vi "FPGA with torque filterMain.vi"() -> ()   [LabVIEW 2018]
doc: "This VI reads all analogue data channels available at the fastest rate supported by the respective hardware and updates a memory address for when each measurement is available.\n\nAt a rate defined by the fastest module (NI 9237 - default of 12.5kHz) this memory is read, combined with the measurements from the 9237 module and written to the FIFO for communication to the RT machine.\n\nThe NI 9237 modeul therefore defines the nominal sampling rate of the system (with slower channels over-sampled).\n\nA time channel (in uSec) is provided with 0 referenced from the first acquisition of the NI 9237 module"
uses:
  <vilib>/LabVIEW Targets/FPGA/cRIO/shared/nicrio_ModuleControls/nicrio_cRIO-9237_DataRatesRing.ctl
  <vilib>/Platform/TimedLoop/XDataNode/timing_clust.ctl
  <vilib>/Platform/TimedLoop/XDataNode/nitl_modes.ctl
  <vilib>/Platform/TimedLoop/XDataNode/wakeup.ctl
  <vilib>/rvi/Emulation/niFpgaGetClockAttributes.vi
  <vilib>/rvi/Emulation/niFpgaSctlEmulationGetInTimedLoop.vi
  <vilib>/rvi/Emulation/niFpgaEmulationReportErrorSimple.vi
  <vilib>/rvi/Emulation/niFpgaProcessEmulError.vi
  <vilib>/rvi/eio/common/nirviEmuTemplatePropertySet_noerrors.vi
  <vilib>/rvi/eio/common/nirviEmuTemplateMethod_errors.vi
  <vilib>/rvi/interface/RandomDataEmulation/niFpgaRandomDataHandleErrors.vi
  <vilib>/rvi/Memory/Memory_Emulation/nirvimemoryFastEmulation.vi
  <vilib>/rvi/Memory/Memory_Emulation/nirvimemoryEmulation.vi
  <vilib>/rvi/Emulation/niFpgaEmulationIsFPGAContextNoSignature.vi
  <vilib>/rvi/DataTransferAndStorage/Container/Common/niFpgaContainerGetUniqueNameForEmu.vi
  <vilib>/rvi/errors/nirviReportUnexpectedCaseInternalError (U32).vi
  <vilib>/rvi/Emulation/niFpgaCriticalErrorInLSC.vi
  <vilib>/eio/EIOPropertyNode/EIOPropertyNode.xnode
  <vilib>/eio/EIONode/EIONode.xnode
  <vilib>/rvi/DataTransferAndStorage/Container/XNode/niFpgaContainer.xnode
  <vilib>/rvi/interface/RandomDataEmulation/nirviRandomDataFpgaReadWriteTemplate.vi
  <vilib>/platform/TimedLoop/XDataNode/XDataNode.xnode
  <vilib>/eio/EIOMethodNode/EIOMethodNode.xnode
  <vilib>/Platform/TimedLoop/XDataNode/XDNodeRunTimeDep.lvlib
  <vilib>/rvi/eio/common/nirviEmuTemplatePropertyGet_errors.vi
  <vilib>/rvi/eio/common/nirviEmuTemplatePropertyGet_noerrors.vi
  <vilib>/rvi/eio/common/nirviEmuTemplatePropertySet_errors.vi
panel:
  in  "Data Rate":T1=1 items=["50.000 kS/s (NI 9237)"=1, "25.000 kS/s (NI 9237)"=2, "16.667 kS/s (NI 9237)"=3, "12.500 kS/s (NI 9237)"=4, "10.000 kS/s (NI 9237)"=5, "8.333 kS/s (NI 9237)"=6, "7.143 kS/s (NI 9237)"=7, "6.250 kS/s (NI 9237)"=8, "5.556 kS/s (NI 9237)"=9, "5.000 kS/s (NI 9237)"=10, "4.545 kS/s (NI 9237)"=11, "4.167 kS/s (NI 9237)"=12, "3.846 kS/s (NI 9237)"=13, "3.571 kS/s (NI 9237)"=14, "3.333 kS/s (NI 9237)"=15, "3.125 kS/s (NI 9237)"=16, "2.941 kS/s (NI 9237)"=17, "2.778 kS/s (NI 9237)"=18, "2.632 kS/s (NI 9237)"=19, "2.500 kS/s (NI 9237)"=20, "2.381 kS/s (NI 9237)"=21, "2.273 kS/s (NI 9237)"=22, "2.174 kS/s (NI 9237)"=23, "2.083 kS/s (NI 9237)"=24, "2.000 kS/s (NI 9237)"=25, "1.923 kS/s (NI 9237)"=26, "1.852 kS/s (NI 9237)"=27, "1.786 kS/s (NI 9237)"=28, "1.724 kS/s (NI 9237)"=29, "1.667 kS/s (NI 9237)"=30, "1.613 kS/s (NI 9237)"=31]
  in  "torque filter":i16=-2
  in  "encoders offset":u32 caption="encoder offset @ 1Hz (ticks)"
  out "Total channel count":u32=61
  out "timestamp":u32
  out "FIFO full counter":i32
  in  "Safe Voltage":fxp<+/-,20,5>[](array[numeric])=[0.0, 0.0, 0.0, 0.0]
  in  "Safe Digital":bool[](array[boolean])=[FALSE, FALSE, FALSE, FALSE, FALSE, FALSE, FALSE, FALSE]
  in  "Voltage Out":fxp<+/-,20,5>[](array[numeric])=[0.0, 0.0, 0.0, 0.0]
  in  "Update Outputs":bool
  in  "Mod 8":bool[](array[boolean])=[FALSE, FALSE, FALSE, FALSE, FALSE, FALSE, FALSE, FALSE]
  out "E Stop":bool
  in  "Stop acquire":bool
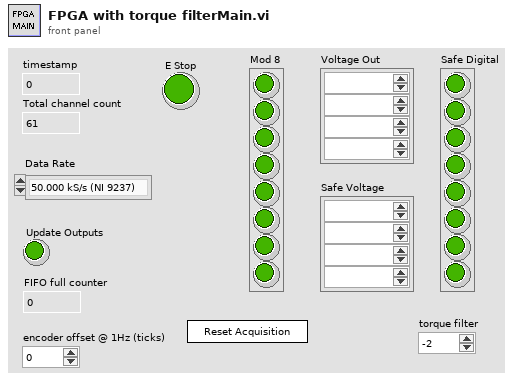
[diagram p1: front panel]
types:
  T1 = typedef "nicrio_cRIO-9237_DataRatesRing.ctl" = u8
  T2 = typedef "XDNodeRunTimeDep.lvlib/timing_clust.ctl" = cluster{"Expected End [f-1]":u64, "Actual End [f-1]":u64, "Finished Late? [f-1]":bool, "Expected End [i-1]":u64, "Actual End [i-1]":u64, "Finished Late? [i-1]":bool, "Expected Start [i]":u64, "Actual Start [i]":u64, "Expected Start [f]":u64, "Actual Start [f]":u64, "Source Name":string, "Structure Name":string, "Period":i64, "Deadline":i64, "Offset":i64, "Start":i64, "Priority":i32, "Timeout":i32, "Mode":T3, "Wakeup Reason":T4, "Error":errorcluster, "Source Type":string, "Secondary Source Type":string, "Global End Time":u64, "Global Start Time":u64, "Frame Duration":u64, "Iteration Duration":u64, "Assigned CPU":i32, "I/O Scan Engine Mode":u32}
  T3 = typedef "XDNodeRunTimeDep.lvlib/nitl_modes.ctl" = enum32{"No Change", "Process missed periods, maintain original phase", "Discard missed periods, maintain original phase", "Process missed periods, ignore original phase", "Discard missed periods, ignore original phase"}
  T4 = typedef "XDNodeRunTimeDep.lvlib/wakeup.ctl" = enum32{"Normal", "Aborted", "Asynchronous wakeup", "Timing source error", "Timed loop error", "Timeout"}
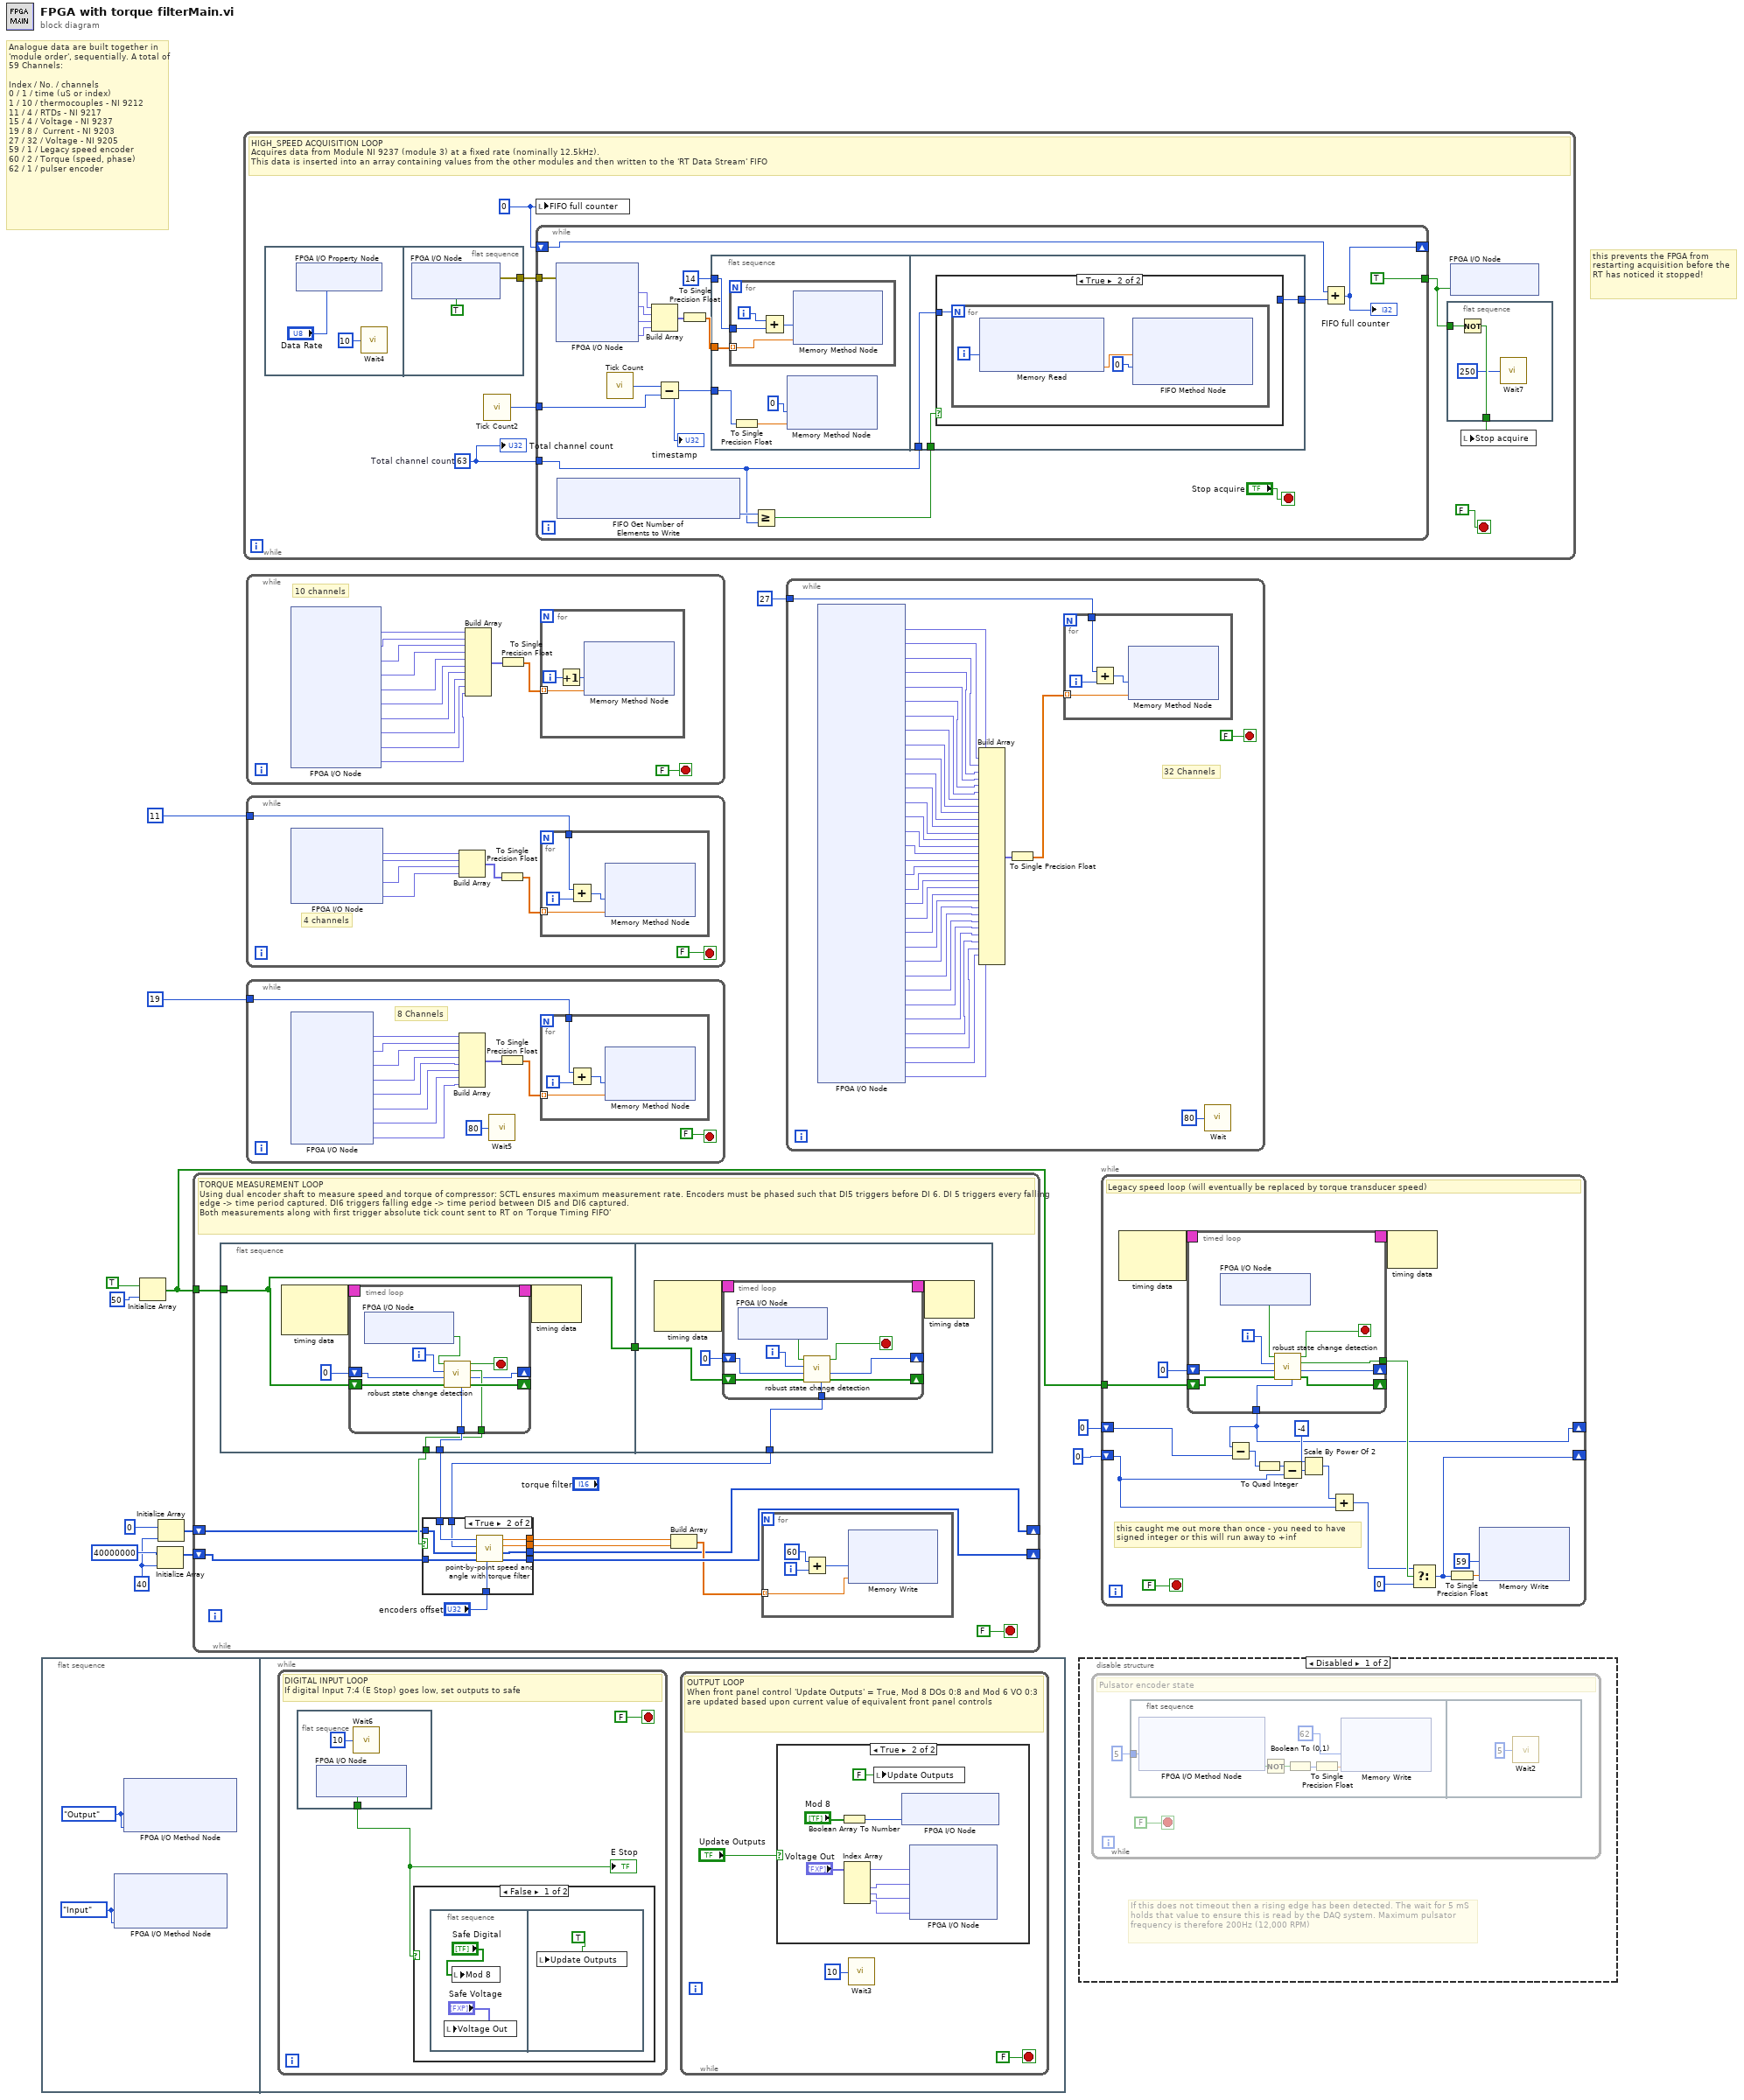
[diagram p0: block diagram]
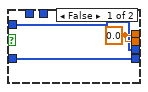
[diagram p5: hidden frame]
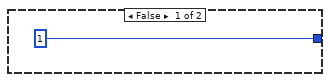
[diagram p6: hidden frame]
diagram:
  w3 = 40 ("dimension size")
  # "this prevents the FPGA from restarting acquisition before the RT has noticed it stopped!"
  # "Analogue data are built together in 'module order', sequentially. A total of 59 Channels:\n\nIndex / No. / channels\n0 / 1 / time (uS or index)\n1 / 10 / thermocouples - NI 9212\n11 / 4 / RTDs - NI 9217\n15 / 4 / Voltage - NI 9237\n19 / 8 /  Current - NI 9203\n27 / 32 / Voltage - NI 9205\n59 / 1 / Legacy speed encoder\n60 / 2 / Torque (speed, phase)\n62 / 1 / pulser encoder"
  n1 = flat-sequence {
    frame #0 {
      w14 = enum8{"No Change", "Input", "Output"}."Output" ("DIO 7:4")
      w15 = enum8{"No Change", "Input", "Output"}."Input" ("DIO 7:4")
      n2 = xnode "FPGA I/O Method Node"("DIO 7:4"=w15, "DIO 3:0"=w15) -> ()  [unwired: 1 in, 1 out]
      n3 = xnode "FPGA I/O Method Node"("DIO 7:4"=w14, "DIO 3:0"=w14) -> ()  [unwired: 1 in, 1 out]
    }
    frame #1 {
      n4 = while {
        stop <- FALSE stop-if-true
        # "DIGITAL INPUT LOOP\nIf digital Input 7:4 (E Stop) goes low, set outputs to safe"
        n5 = flat-sequence {
          tunnel: [w30] -> w27
          frame #0 {
            n6 = xnode "FPGA I/O Node"() -> ("Mod7/DIO4"=w30:bool)  [unwired: 1 in, 1 out]
            n7 = call "Wait6"("Count(uSec)"=u8 10) -> ()  [unwired: 1 out]
          }
        }
        n8 = case shown="False" w27 {
          frame False {
            n9 = flat-sequence {
              frame #0 {
                n10 = local write "Voltage Out"("Safe Voltage") -> ()
                n11 = local write "Mod 8"("Safe Digital") -> ()
              }
              frame #1 {
                n12 = local write "Update Outputs"(TRUE ("Update Outputs")) -> ()
              }
            }
          }
          frame True {
          }
        }
        "E Stop" <- w27
      }
      n13 = while {
        stop <- FALSE stop-if-true
        # "OUTPUT LOOP\nWhen front panel control 'Update Outputs' = True, Mod 8 DOs 0:8 and Mod 6 VO 0:3 are updated based upon current value of equivalent front panel controls"
        n14 = case shown="True" "Update Outputs" {
          frame False {
          }
          frame True {
            n15 = Boolean Array To Number(Boolean array="Mod 8") -> (number=w25:u8)
            n16 = Index Array(array="Voltage Out") -> (element #1=w23:fxp<+/-,20,5>, element #2=w22:fxp<+/-,20,5>, element #3=w21:fxp<+/-,20,5>, element #4=w20:fxp<+/-,20,5>)  [unwired: 4 in]
            n17 = local write "Update Outputs"(FALSE ("Update Outputs")) -> ()
            n18 = xnode "FPGA I/O Node"("Mod8/DIO7:0"=w25) -> ()  [unwired: 1 in, 1 out]
            n19 = xnode "FPGA I/O Node"("Mod6/AO0"=w23, "Mod6/AO1"=w22, "Mod6/AO2"=w21, "Mod6/AO3"=w20) -> ()  [unwired: 4 in, 4 out]
          }
        }
        n20 = call "Wait3"("Count(uSec)"=u16 10 ("Count(Ticks)")) -> ()  [unwired: 1 out]
      }
    }
  }
  n21 = Initialize Array(TRUE, 50 ("edge buffer size")) -> (w5:bool[])
  n22 = Initialize Array(u32 40000000 ("64bit integer"), w3) -> (w8:u32[])
  n23 = Initialize Array(0 ("64bit integer"), w3) -> (w1:i32[])
  n24 = while {
    shift-right: [w43] -> _
    shift-left: w8 -> [w44]
    tunnel: w5 -> [w38]
    shift-right: [w35] -> _
    shift-left: w1 -> [w36]
    stop <- FALSE stop-if-true
    # "TORQUE MEASUREMENT LOOP\nUsing dual encoder shaft to measure speed and torque of compressor: SCTL ensures maximum measurement rate. Encoders must be phased such that DI5 triggers before DI 6. DI 5 triggers every falling edge -> time period captured. DI6 triggers falling edge -> time period between DI5 and DI6 captured.\nBoth measurements along with first trigger absolute tick count sent to RT on 'Torque Timing FIFO'"
    n25 = flat-sequence {
      tunnel: [w67] -> w46
      tunnel: [w66] -> w39
      tunnel: w38 -> [w64]
      tunnel: [w64] -> w37
      tunnel: [w87] -> w45
      tunnel: w37 -> [w86]
      frame #0 {
        n26 = node-c288() -> (w69:T2)  [unwired: 2 in]
        n27 = timed-loop {
          timing: w69 -> [_]
          timing-out: [_] -> w68
          tunnel: [w73] -> w67
          tunnel: [w72] -> w66
          shift-right: [w76] -> _
          shift-left: w64 -> [w77]
          shift-right: [w70] -> _
          shift-left: i16 0 ("step") -> [w74]
          i -> [w75]
          stop <- w71 stop-if-true
          n28 = xnode "FPGA I/O Node"() -> ("Mod7/DIO0"=w78:bool)  [unwired: 1 in, 1 out]
          n29 = call "robust state change detection.vi"("history"=w77, "step"=w74, "tick"=w75, "New state"=w78) -> ("history out"=w76:bool[], "step out"=w70:i16, "edge detected"=w72:bool, "Stop?"=w71:bool, "tick"=w73:u32)  [unwired: 3 in]
        }
        n30 = node-c288(w68) -> ()  [unwired: 1 out]
      }
      frame #1 {
        n31 = node-c288() -> (w85:T2)  [unwired: 2 in]
        n32 = timed-loop {
          timing: w85 -> [_]
          timing-out: [_] -> w84
          shift-right: [w93] -> _
          shift-left: w86 -> [w94]
          tunnel: [w91] -> w87
          shift-right: [w88] -> _
          shift-left: i16 0 ("step") -> [w89]
          i -> [w90]
          stop <- w92 stop-if-true
          n33 = xnode "FPGA I/O Node"() -> ("Mod7/DIO1"=w95:bool)  [unwired: 1 in, 1 out]
          n34 = call "robust state change detection.vi"("history"=w94, "step"=w89, "tick"=w90, "New state"=w95) -> ("history out"=w93:bool[], "step out"=w88:i16, "Stop?"=w92:bool, "tick"=w91:u32)  [unwired: 3 in, 1 out]
        }
        n35 = node-c288(w84) -> ()  [unwired: 1 out]
      }
    }
    n36 = case shown="True" w39 {
      tunnel: w46 -> [_ w59]
      tunnel: w45 -> [_ w58]
      tunnel: w44 -> [w50 w57]
      tunnel: [w50 w56] -> w43
      tunnel: "encoders offset" -> [_ w55]
      tunnel: [w49 w54] -> w41
      tunnel: [w49 w53] -> w34
      tunnel: w36 -> [w48 w52]
      tunnel: [w48 w51] -> w35
      frame False {
        w49 = sgl 0.0 ("calculated speed (Hz)")
      }
      frame True {
        n37 = call "point-by-point speed and angle with torque filter.vi"("encoders offset"=w55, "speed history in"=w57, "torque history"=w52, "angle pulse"=w58, "speed pulse"=w59) -> ("speed history out"=w56:u32[], "torque history out"=w51:i32[], "calculated angle (degrees)"=w53:sgl, "calculated speed (Hz)"=w54:sgl)  [unwired: 2 in, 1 out]
      }
    }
    n38 = Build Array(w41, w34) -> (w40:sgl[])
    n39 = for {
      tunnel: w40 -> [w60] mode=indexing
      i -> [w61]
      n40 = Add(x=u32 60 ("Address"), y=w61) -> (x+y=w62:u32)
      n41 = xnode ("Memory Write")("Address"=w62, "Data"=w60) -> ()  [unwired: 1 in, 1 out]
    }
  }
  n42 = while {
    stop <- FALSE stop-if-true
    w101 = 0 ("FIFO full counter")
    w104 = u32 63  # Total channel count
    # "HIGH_SPEED ACQUISITION LOOP\nAcquires data from Module NI 9237 (module 3) at a fixed rate (nominally 12.5kHz).\nThis data is inserted into an array containing values from the other modules and then written to the 'RT Data Stream' FIFO"
    n43 = flat-sequence {
      tunnel: [w113] -> w105
      frame #0 {
        n44 = xnode "FPGA I/O Property Node"("Data Rate"="Data Rate") -> ()  [unwired: 1 in, 1 out]
        n45 = call "Wait4"("Count(mSec)"=u16 10) -> ()  [unwired: 1 out]
      }
      frame #1 {
        n46 = xnode "FPGA I/O Node"("Mod3/Start"=TRUE) -> ("error out"=w113:errorcluster)  [unwired: 2 in, 1 out]
      }
    }
    n47 = call "Tick Count2"() -> ("Tick Count(uSec)"=w106:u32)
    n48 = local write "FIFO full counter"(w101) -> ()
    n49 = while {
      tunnel: [TRUE ("I/O Item")] -> w103
      tunnel: w105 -> [w131]
      tunnel: w104 -> [w116]
      shift-right: [w124] -> _
      shift-left: w101 -> [w122]
      tunnel: w106 -> [w125]
      stop <- "Stop acquire" stop-if-true
      n50 = xnode "FPGA I/O Node"("error in"=w131) -> ("Mod3/AI0"=w130:fxp<+/-,24,-4>, "Mod3/AI1"=w129:fxp<+/-,24,-4>, "Mod3/AI2"=w128:fxp<+/-,24,-4>, "Mod3/AI3"=w127:fxp<+/-,24,-4>)  [unwired: 4 in, 5 out]
      n51 = xnode ("FIFO Get Number of Elements to Write")() -> ("Number of Elements to Write"=w118:u32)  [unwired: 1 in, 1 out]
      n52 = call "Tick Count"() -> ("Tick Count(uSec)"=w121:u32)
      n53 = Build Array(w130, w129, w128, w127) -> (w126:fxp<+/-,24,-4>[])
      n54 = Subtract(x=w121, y=w125) -> (x-y=w114:u32)
      "timestamp" <- w114
      n55 = To Single Precision Float(number=w126) -> (single precision float=w120:sgl[])
      n56 = flat-sequence {
        tunnel: w120 -> [w137]
        tunnel: 14 ("index") -> [w136]
        tunnel: w114 -> [w134]
        tunnel: w116 -> [w144]
        tunnel: [w143] -> w115
        tunnel: w117 -> [w142]
        frame #0 {
          n57 = for {
            tunnel: w137 -> [w141] mode=indexing
            tunnel: w136 -> [w140]
            i -> [w138]
            n58 = Add(x=w138, y=w140) -> (x+y=w139:i32)
            n59 = xnode ("Memory Method Node")("Address"=w139, "Data"=w141) -> ()  [unwired: 1 in, 1 out]
          }
          n60 = To Single Precision Float(number=w134) -> (single precision float=w135:sgl)
          n61 = xnode ("Memory Method Node")("Address"=u32 0, "Data"=w135) -> ()  [unwired: 1 in, 1 out]
        }
        frame #1 {
          n62 = case shown="True" w142 {
            tunnel: [1 _] -> w143
            tunnel: w144 -> [_ w146]
            frame False {
            }
            frame True {
              n63 = for {
                N: w146 -> [_]
                i -> [w147]
                n64 = xnode ("Memory Read")("Address"=w147) -> ("Data"=w148:sgl)  [unwired: 1 in, 1 out]
                n65 = xnode ("FIFO Method Node")("Element"=w148, "Timeout"=0) -> ()  [unwired: 1 in, 2 out]
              }
            }
          }
        }
      }
      n66 = Greater Or Equal?(x=w118, y=w116) -> (x >= y?=w117:bool)
      n67 = Add(x=w122, y=w115) -> (x+y=w124:i32)
      "FIFO full counter" <- w124
    }
    n68 = flat-sequence {
      tunnel: w103 -> [w109]
      tunnel: [w108] -> w100
      frame #0 {
        n69 = Not(x=w109) -> (.not. x?=w108:bool)
        n70 = call "Wait7"("Count(mSec)"=u8 250) -> ()  [unwired: 1 out]
      }
    }
    n71 = xnode "FPGA I/O Node"("Mod3/Stop"=w103) -> ()  [unwired: 1 in, 1 out]
    n72 = local write "Stop acquire"(w100) -> ()
    "Total channel count" <- w104
  }
  n73 = while {
    stop <- FALSE stop-if-true
    # "10 channels"
    n74 = xnode "FPGA I/O Node"() -> ("Mod1/TC0"=w162:fxp<+/-,24,-2>, "Mod1/TC1"=w161:fxp<+/-,24,-2>, "Mod1/TC2"=w160:fxp<+/-,24,-2>, "Mod1/TC3"=w159:fxp<+/-,24,-2>, "Mod1/TC4"=w158:fxp<+/-,24,-2>, "Mod1/TC5"=w157:fxp<+/-,24,-2>, "Mod1/TC6"=w156:fxp<+/-,24,-2>, "Mod1/TC7"=w155:fxp<+/-,24,-2>, "Mod1/CJC0"=w152:fxp<+/-,24,-2>, "Mod1/CJC1"=w151:fxp<+/-,24,-2>)  [unwired: 10 in, 10 out]
    n75 = Build Array(w162, w161, w160, w159, w158, w157, w156, w155, w152, w151) -> (w154:fxp<+/-,24,-2>[])
    n76 = To Single Precision Float(number=w154) -> (single precision float=w153:sgl[])
    n77 = for {
      tunnel: w153 -> [w165] mode=indexing
      i -> [w164]
      n78 = Increment(x=w164) -> (x+1=w163:i32)
      n79 = xnode ("Memory Method Node")("Address"=w163, "Data"=w165) -> ()  [unwired: 1 in, 1 out]
    }
  }
  n80 = while {
    tunnel: 11 ("Numeric") -> [w167]
    stop <- FALSE stop-if-true
    # "4 channels"
    n81 = xnode "FPGA I/O Node"() -> ("Mod2/RTD0"=w173:fxp<+/-,24,10>, "Mod2/RTD1"=w172:fxp<+/-,24,10>, "Mod2/RTD2"=w171:fxp<+/-,24,10>, "Mod2/RTD3"=w168:fxp<+/-,24,10>)  [unwired: 4 in, 4 out]
    n82 = Build Array(w173, w172, w171, w168) -> (w170:fxp<+/-,24,10>[])
    n83 = To Single Precision Float(number=w170) -> (single precision float=w169:sgl[])
    n84 = for {
      tunnel: w169 -> [w177] mode=indexing
      tunnel: w167 -> [w174]
      i -> [w176]
      n85 = Add(x=w174, y=w176) -> (x+y=w175:i32)
      n86 = xnode ("Memory Method Node")("Address"=w175, "Data"=w177) -> ()  [unwired: 1 in, 1 out]
    }
  }
  n87 = while {
    tunnel: 19 ("Numeric") -> [w184]
    stop <- FALSE stop-if-true
    # "8 Channels"
    n88 = xnode "FPGA I/O Node"() -> ("Mod4/AI0"=w190:fxp<+/-,21,-4>, "Mod4/AI1"=w189:fxp<+/-,21,-4>, "Mod4/AI2"=w188:fxp<+/-,21,-4>, "Mod4/AI3"=w185:fxp<+/-,21,-4>, "Mod4/AI4"=w183:fxp<+/-,21,-4>, "Mod4/AI5"=w182:fxp<+/-,21,-4>, "Mod4/AI6"=w181:fxp<+/-,21,-4>, "Mod4/AI7"=w180:fxp<+/-,21,-4>)  [unwired: 8 in, 8 out]
    n89 = Build Array(w190, w189, w188, w185, w183, w182, w181, w180) -> (w187:fxp<+/-,21,-4>[])
    n90 = call "Wait5"("Count(uSec)"=u8 80) -> ()  [unwired: 1 out]
    n91 = To Single Precision Float(number=w187) -> (single precision float=w186:sgl[])
    n92 = for {
      tunnel: w186 -> [w194] mode=indexing
      tunnel: w184 -> [w191]
      i -> [w193]
      n93 = Add(x=w191, y=w193) -> (x+y=w192:i32)
      n94 = xnode ("Memory Method Node")("Address"=w192, "Data"=w194) -> ()  [unwired: 1 in, 1 out]
    }
  }
  n95 = while {
    tunnel: 27 ("Numeric") -> [w230]
    stop <- FALSE stop-if-true
    # "32 Channels"
    n96 = xnode "FPGA I/O Node"() -> ("Mod5/AI0"=w198:fxp<+/-,26,5>, "Mod5/AI1"=w199:fxp<+/-,26,5>, "Mod5/AI2"=w200:fxp<+/-,26,5>, "Mod5/AI3"=w201:fxp<+/-,26,5>, "Mod5/AI4"=w202:fxp<+/-,26,5>, "Mod5/AI5"=w203:fxp<+/-,26,5>, "Mod5/AI6"=w204:fxp<+/-,26,5>, "Mod5/AI7"=w205:fxp<+/-,26,5>, "Mod5/AI8"=w229:fxp<+/-,26,5>, "Mod5/AI9"=w228:fxp<+/-,26,5>, "Mod5/AI10"=w227:fxp<+/-,26,5>, "Mod5/AI11"=w226:fxp<+/-,26,5>, "Mod5/AI12"=w225:fxp<+/-,26,5>, "Mod5/AI13"=w224:fxp<+/-,26,5>, "Mod5/AI14"=w223:fxp<+/-,26,5>, "Mod5/AI15"=w222:fxp<+/-,26,5>, "Mod5/AI16"=w221:fxp<+/-,26,5>, "Mod5/AI17"=w220:fxp<+/-,26,5>, "Mod5/AI18"=w219:fxp<+/-,26,5>, "Mod5/AI19"=w218:fxp<+/-,26,5>, "Mod5/AI20"=w217:fxp<+/-,26,5>, "Mod5/AI21"=w216:fxp<+/-,26,5>, "Mod5/AI22"=w215:fxp<+/-,26,5>, "Mod5/AI23"=w214:fxp<+/-,26,5>, "Mod5/AI24"=w213:fxp<+/-,26,5>, "Mod5/AI25"=w212:fxp<+/-,26,5>, "Mod5/AI26"=w211:fxp<+/-,26,5>, "Mod5/AI27"=w210:fxp<+/-,26,5>, "Mod5/AI28"=w209:fxp<+/-,26,5>, "Mod5/AI29"=w208:fxp<+/-,26,5>, "Mod5/AI30"=w207:fxp<+/-,26,5>, "Mod5/AI31"=w206:fxp<+/-,26,5>)  [unwired: 32 in, 32 out]
    n97 = Build Array(w198, w199, w200, w201, w202, w203, w204, w205, w229, w228, w227, w226, w225, w224, w223, w222, w221, w220, w219, w218, w217, w216, w215, w214, w213, w212, w211, w210, w209, w208, w207, w206) -> (w231:fxp<+/-,26,5>[])
    n98 = To Single Precision Float(number=w231) -> (single precision float=w197:sgl[])
    n99 = for {
      tunnel: w197 -> [w235] mode=indexing
      tunnel: w230 -> [w232]
      i -> [w234]
      n100 = Add(x=w232, y=w234) -> (x+y=w233:i32)
      n101 = xnode ("Memory Method Node")("Address"=w233, "Data"=w235) -> ()  [unwired: 1 in, 1 out]
    }
    n102 = call "Wait"("Count(uSec)"=u8 80) -> ()  [unwired: 1 out]
  }
  n103 = disable-structure shown="Disabled" {
    frame Disabled {
      # "If this does not timeout then a rising edge has been detected. The wait for 5 mS holds that value to ensure this is read by the DAQ system. Maximum pulsator frequency is therefore 200Hz (12,000 RPM)"
      n104 = while {
        stop <- FALSE stop-if-true
        # "Pulsator encoder state"
        n105 = flat-sequence {
          tunnel: 5 ("Timeout") -> [w240]
          frame #0 {
            n106 = xnode "FPGA I/O Method Node"("Timeout"=w240) -> ("Timed Out"=w239:bool)  [unwired: 1 in, 1 out]
            n107 = Not(x=w239) -> (.not. x?=w238:bool)
            n108 = Boolean To (0,1)(Boolean=w238) -> (0, 1=w243:i16)
            n109 = To Single Precision Float(number=w243) -> (single precision float=w242:sgl)
            n110 = xnode ("Memory Write")("Address"=u32 62, "Data"=w242) -> ()  [unwired: 1 in, 1 out]
          }
          frame #1 {
            n111 = call "Wait2"("Count(mSec)"=u16 5 ("Count(uSec)")) -> ()  [unwired: 1 out]
          }
        }
      }
    }
    frame Enabled {
    }
  }
  n112 = while {
    shift-right: [w250] -> _
    shift-left: i64 0 -> [w257]
    tunnel: w5 -> [w251]
    shift-right: [w246] -> _
    shift-left: u32 0 ("tick") -> [w245]
    stop <- FALSE stop-if-true
    # "this caught me out more than once - you need to have signed integer or this will run away to +inf"
    # "Legacy speed loop (will eventually be replaced by torque transducer speed)"
    n113 = node-c288() -> (w263:T2)  [unwired: 2 in]
    n114 = timed-loop {
      timing: w263 -> [_]
      timing-out: [_] -> w262
      shift-right: [w269] -> _
      shift-left: i16 0 ("step") -> [w270]
      tunnel: [w267] -> w252
      tunnel: [w266] -> w246
      shift-right: [w264] -> _
      shift-left: w251 -> [w265]
      i -> [w271]
      stop <- w268 stop-if-true
      n115 = xnode "FPGA I/O Node"() -> ("Mod7/DIO3"=w272:bool)  [unwired: 1 in, 1 out]
      n116 = call "robust state change detection.vi"("history"=w265, "step"=w270, "tick"=w271, "New state"=w272) -> ("history out"=w264:bool[], "step out"=w269:i16, "edge detected"=w267:bool, "Stop?"=w268:bool, "tick"=w266:u32)  [unwired: 3 in]
    }
    n117 = Subtract(x=w246, y=w245) -> (x-y=w247:u32)
    n118 = To Quad Integer(1:w247) -> (0:w254:i64)
    n119 = Subtract(x=w254, y=w257) -> (x-y=w258:i64)
    n120 = Scale By Power Of 2(n=i16 -4, x=w258) -> (x*2^n=w260:i64)
    n121 = Add(x=w260, y=w257) -> (x+y=w248:i64)
    n122 = node-c288(w262) -> ()  [unwired: 1 out]
    n123 = Select(t=w248, s=w252, f=u32 0 ("t")) -> (s? t:f=w250:i64)
    n124 = To Single Precision Float(number=w250) -> (single precision float=w256:sgl)
    n125 = xnode ("Memory Write")("Address"=u32 59, "Data"=w256) -> ()  [unwired: 1 in, 1 out]
  }
